vi "String Index.vi"(2 "String Array":string[](array[string]), 3 "search string":string) -> (0 "error":i32, 1 "index":i32)   [LabVIEW 2024, in "NI_Gmath.lvlib"]
uses:
  NI_Gmath.lvlib
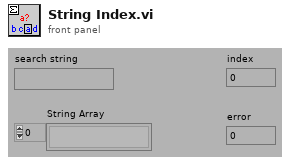
[diagram p1: front panel]
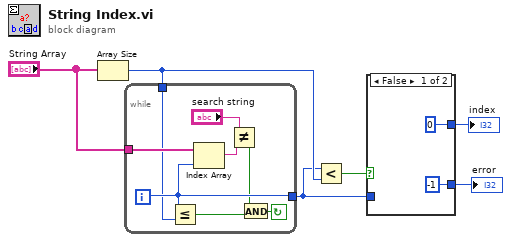
[diagram p0: block diagram]
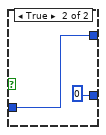
[diagram p2: hidden frame]
diagram:
  n1 = Array Size(array="String Array") -> (size(s)=w5:i32)
  n2 = while {
    tunnel: [w10] -> w2
    tunnel: "String Array" -> [w14]
    tunnel: w5 -> [w9]
    i -> [w10]
    stop <- w8 continue-if-true
    n3 = Less Or Equal?(x=w10, y=w9) -> (x <= y?=w11:bool)
    n4 = Index Array(array=w14, index=w10) -> (element=w12:string)
    n5 = Not Equal?(x="search string", y=w12) -> (x != y?=w7:bool)
    n6 = And(x=w7, y=w11) -> (x .and. y?=w8:bool)
  }
  n7 = Less?(x=w2, y=w5) -> (x < y?=w4:bool)
  n8 = case shown="False" w4 {
    tunnel: [-1 0] -> w3
    tunnel: w2 -> [_ w18]
    tunnel: [0 w18] -> w1
    frame False {
    }
    frame True {
    }
  }
  "error" <- w3
  "index" <- w1
